vi "GaussianFilter.vi"(2 "Order (width)":i32, 3 "X":dbl[](array[numeric])) -> (0 "Filter Coefficients":dbl[](array[numeric]), 1 "Filtered X":dbl[](array[numeric]))   [LabVIEW 2019, in "Nanonis Prog Interface.lvlib"]
uses:
  <userlib>/Nanonis Prog Interface V5/Nanonis Prog Interface.lvlib
  <vilib>/Analysis/baseanly.llb/Real Dot Product.vi
  <vilib>/Analysis/NI_AALBase.lvlib
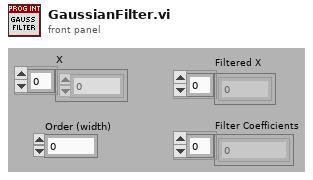
[diagram p1: front panel]
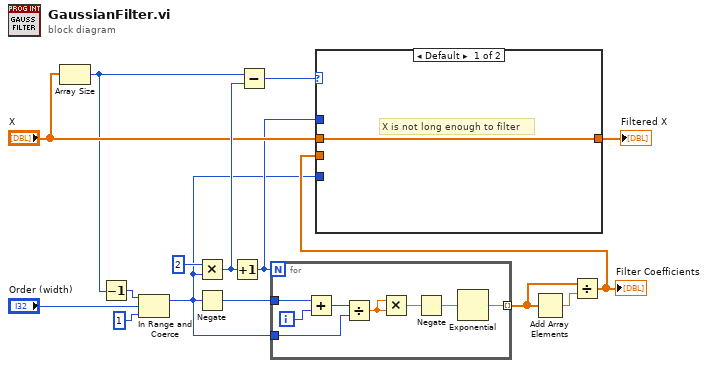
[diagram p0: block diagram]
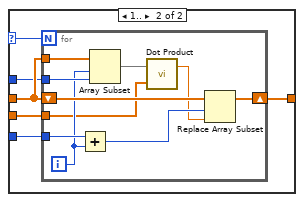
[diagram p2: hidden frame]
diagram:
  n1 = Array Size(array="X") -> (size(s)=w2:i32)
  n2 = Decrement(x=w2) -> (x-1=w3:i32)
  n3 = In Range and Coerce(upper limit=w3, x="Order (width)", lower limit=1) -> (coerced(x)=w4:i32)  [unwired: 1 out]
  n4 = Multiply(x=2 ("y"), y=w4) -> (x*y=w11:i32)
  n5 = Negate(x=w4) -> (-x=w15:i32)
  n6 = Increment(x=w11) -> (x+1=w7:i32)
  n7 = Subtract(x=w2, y=w11) -> (x-y=w10:i32)
  n8 = for {
    N: w7 -> [_]
    tunnel: w15 -> [w22]
    tunnel: w4 -> [w20]
    tunnel: [w16] -> w14 mode=indexing
    i -> [w23]
    n9 = Add(x=w22, y=w23) -> (x+y=w21:i32)
    n10 = Divide(x=w21, y=w20) -> (x/y=w19:dbl)
    n11 = Multiply(x=w19, y=w19) -> (x*y=w18:dbl)
    n12 = Negate(x=w18) -> (-x=w17:dbl)
    n13 = Exponential(1:w17) -> (0:w16:dbl)
  }
  n14 = Add Array Elements(numeric array=w14) -> (sum=w13:dbl)
  n15 = Divide(x=w14, y=w13) -> (x/y=w6:dbl[])
  "Filter Coefficients" <- w6
  n16 = case shown="Default" w10 {
    selector: w10 -> [_ w28]
    tunnel: "X" -> [w24 w29]
    tunnel: [w24 w30] -> w9
    tunnel: w4 -> [_ w27]
    tunnel: w7 -> [_ w26]
    tunnel: w6 -> [_ w25]
    frame Default {
      # "X is not long enough to filter"
    }
    frame 1.. {
      n17 = for {
        N: w28 -> [_]
        tunnel: w29 -> [w40]
        shift-right: [w37] -> w30
        shift-left: w29 -> [w38]
        tunnel: w27 -> [w39]
        tunnel: w26 -> [w36]
        tunnel: w25 -> [w31]
        i -> [w35]
        n18 = Add(x=w39, y=w35) -> (x+y=w33:i32)
        n19 = Array Subset(array=w40, index=w35, length=w36) -> (w34:dbl[])
        n20 = call-poly <vilib>:"Dot Product.vi"("Y Vector"=w31, "X Vector"=w34) -> ("X * Y"=w32:dbl)  [unwired: 1 out]
        n21 = Replace Array Subset(array=w38, new element=w32, index=w33) -> (w37:dbl[])
      }
    }
  }
  "Filtered X" <- w9
